vi "Calibrate.vi"(8 "error in (no error)":errorcluster, 11 "VISA resource name":refnum<visa-resource-name>) -> (0 "error out":errorcluster, 2 "Result":i32, 3 "VISA resource name out":refnum<visa-resource-name>)   [LabVIEW 2019, in "Yokogawa WT300 Series.lvlib"]
doc: "Zero-level compensation is the process of creating a zero-input condition using the WT300 internal circuit and setting the level at that point to the zero level. It must be performed to meet the specifications of this instrument."
uses:
  Yokogawa WT300 Series.lvlib
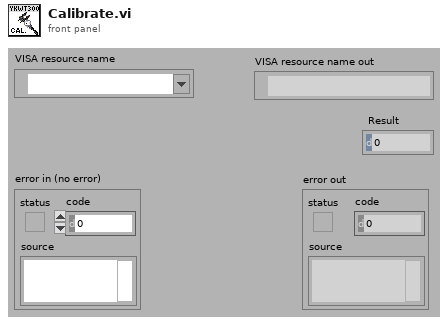
[diagram p1: front panel]
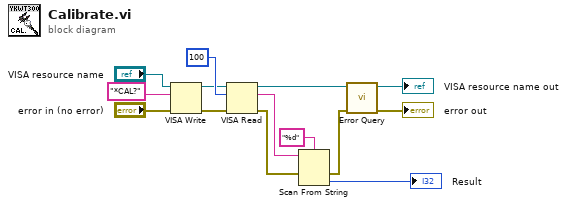
[diagram p0: block diagram]
diagram:
  n1 = VISA Write ("VISA書き込み")(VISA resource name="VISA resource name", write buffer="*CAL?", error in (no error)="error in (no error)") -> (VISA resource name out=w8:refnum<visa-resource-name>, error out=w7:errorcluster)  [unwired: 1 out]
  n2 = VISA Read ("VISA読み取り")(VISA resource name=w8, byte count=u32 100, error in (no error)=w7) -> (VISA resource name out=w6:refnum<visa-resource-name>, read buffer=w4:string, error out=w5:errorcluster)  [unwired: 1 out]
  n3 = Scan From String ("文字列からスキャン")(format string="%d", input string=w4, error in=w5) -> (error out=w2:errorcluster, output 1=→"Result":i32)  [unwired: 2 in, 2 out]
  n4 = call "Error Query.vi"("error in (no error)"=w2, "VISA resource name"=w6) -> ("error out"=→"error out":errorcluster, "VISA resource name out"=→"VISA resource name out":refnum<visa-resource-name>)  [unwired: 6 in, 2 out]
